vi "Modbus Samsung.vi"(5 "address":string, 6 "# Racks":i32=1, 7 "port (502)":u16=502, 8 "Error In":errorcluster, 10 "ES Reset":bool=TRUE, 11 "ES ON Array":bool[](array[boolean])) -> (0 "Error Out":errorcluster, 1 "Current Limit Parameters Out":T5 {"Min Cell Voltage Actual Value" format="%#.2f"; "Max Cell Voltage Actual Value" format="%#.2f"}, 2 "Energy Storage String Data Out":T3, 3 "Energy Storage System Data Out":T1={"Voltage"=0.0, "Current"=0.0, "SOC Avg"=0.0, "Faults"=0, "Alarms"=0, "# Strings"=0, "Max Temp"=0, "Min Temp"=0, "Max Cell Voltage"=0.0, "Min Cell Voltage"=0.0, "Energy Capacity"=0.0, "Energy Remaining"=0.0, "SOC Min"=0.0, "SOC Max"=0.0, "ES Fault"=FALSE, "String Select"=enum."3 Strings", "ES Com Fault"=FALSE, "SOH Avg"=0.0}, 4 "TCP Master Ref Out":refnum<class "Modbus Master.lvclass">)   [LabVIEW 2014]
uses:
  Controls/ModbusState.ctl
  <vilib>/Modbus/master/Modbus Master.lvclass
  Controls/Current Limit Parameters.ctl
  Controls/ES String Array.ctl
  Controls/ES String Data.ctl
  Controls/ES System Data.ctl
  Controls/StringSelector.ctl
  <vilib>/Modbus/master/Create Master Instance (TCP).vi
panel:
  out "Modbus State Out":T6
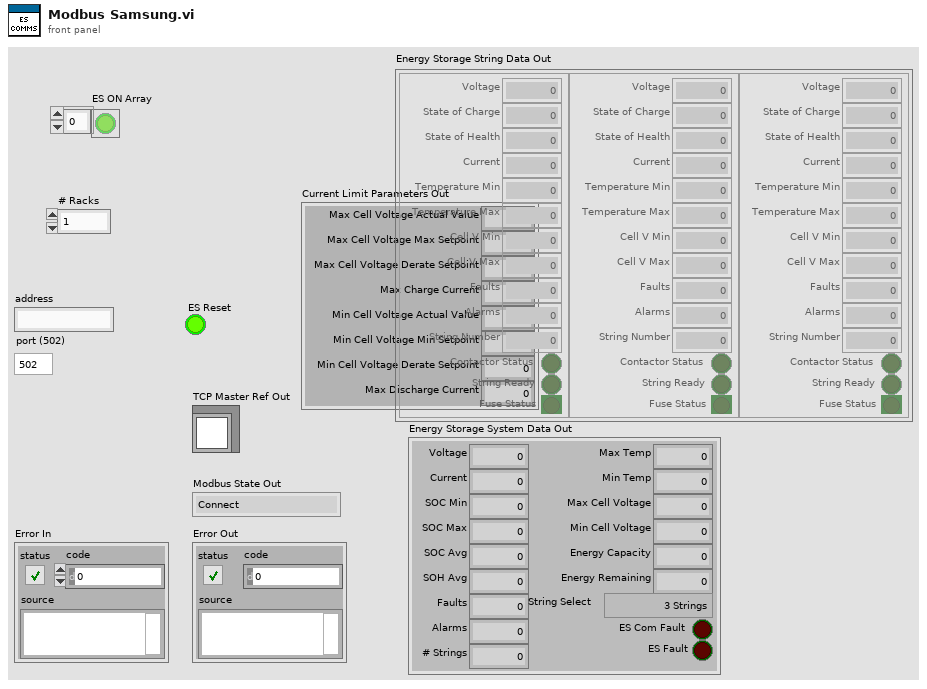
[diagram p1: front panel]
types:
  T1 = typedef "ES System Data.ctl" = cluster{"Voltage":sgl, "Current":sgl, "SOC Avg":sgl, "Faults":u16, "Alarms":u16, "# Strings":u16, "Max Temp":i16, "Min Temp":i16, "Max Cell Voltage":sgl, "Min Cell Voltage":sgl, "Energy Capacity":sgl, "Energy Remaining":sgl, "SOC Min":sgl, "SOC Max":sgl, "ES Fault":bool, "String Select":T2, "ES Com Fault":bool, "SOH Avg":sgl}
  T2 = typedef "StringSelector.ctl" = enum16{"1 String (1)", "1 String (2)", "1 String (3)", "2 Strings (1 2)", "2 Strings (2 3)", "2 Strings (1 3)", "3 Strings"}
  T3 = typedef "ES String Array.ctl" = T4[]
  T4 = typedef "ES String Data.ctl" = cluster{"Voltage":sgl, "State of Charge":sgl, "Current":sgl, "Temperature Min":i16, "Temperature Max":i16, "Faults":u16, "Alarms":u16, "String Number":u16, "Contactor Status":bool, "String Ready":bool, "Fuse Status":bool, "Cell V Max":dbl, "Cell V Min":dbl, "State of Health":sgl}
  T5 = typedef "Current Limit Parameters.ctl" = cluster{"Max Cell Voltage Max Setpoint":dbl, "Max Cell Voltage Actual Value":dbl, "Max Cell Voltage Derate Setpoint":dbl, "Max Charge Current":dbl, "Min Cell Voltage Min Setpoint":dbl, "Min Cell Voltage Actual Value":dbl, "Min Cell Voltage Derate Setpoint":dbl, "Max Discharge Current":dbl}
  T6 = typedef "ModbusState.ctl" = enum16{"Connect", "Disconnect", "Set Basic Objects", "Get Basic Objects", "Read", "Write", "Read/Write"}
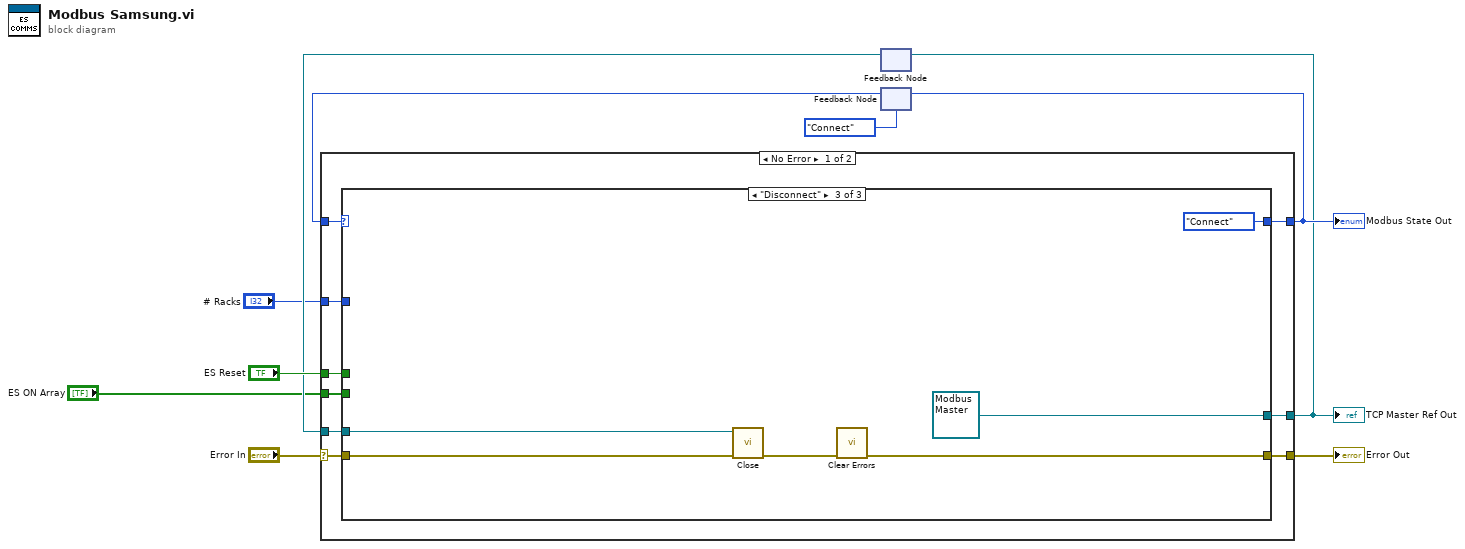
[diagram p0: block diagram]
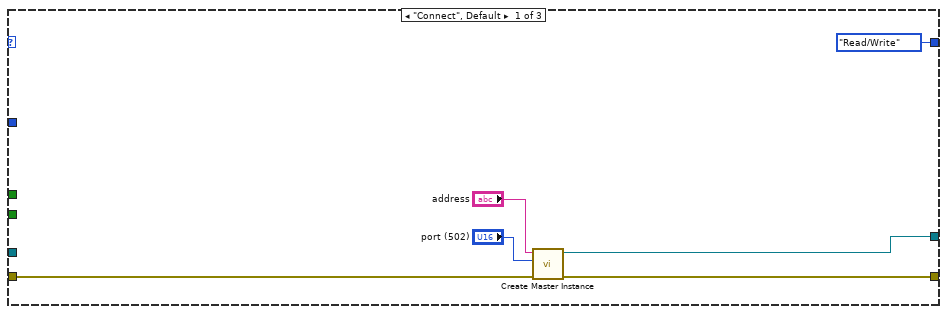
[diagram p2: hidden frame]
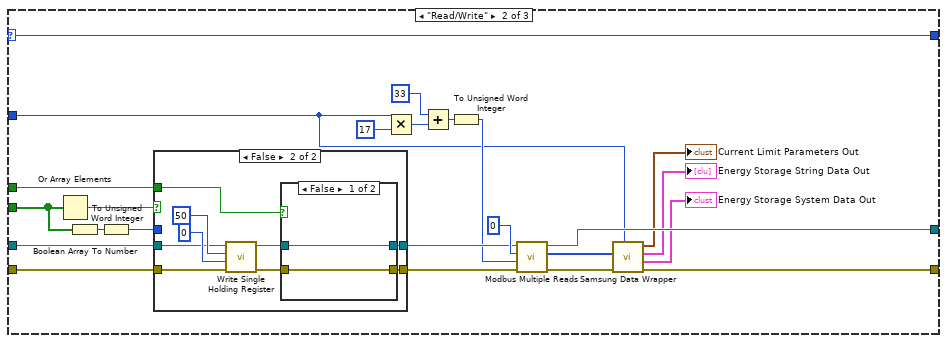
[diagram p3: hidden frame]
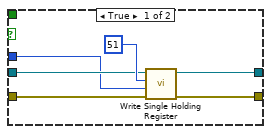
[diagram p4: hidden frame]
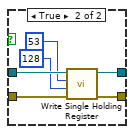
[diagram p5: hidden frame]
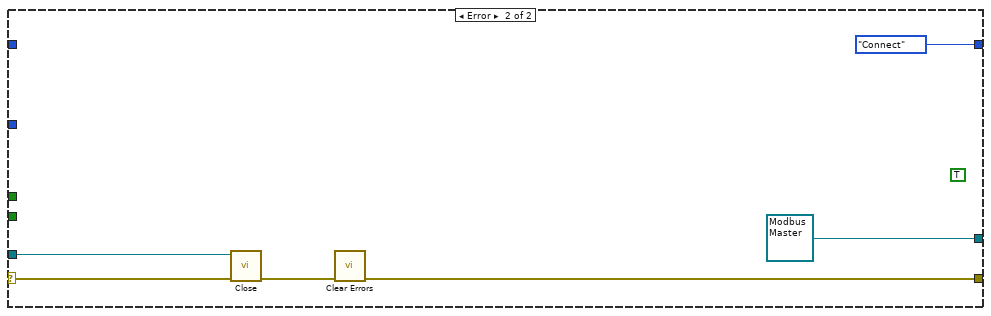
[diagram p6: hidden frame]
diagram:
  n1 = feedback #1() -> (w3:refnum<class "Modbus Master.lvclass">)  [unwired: 1 in]
  n2 = feedback #2(ModbusState."Connect" ("Modbus State In")) -> (w5:T6)
  n3 = case shown="No Error" "Error In" {
    selector: "Error In" -> [w18 w80]
    tunnel: [w15 w79] -> w9
    tunnel: w5 -> [w19 _]
    tunnel: [w17 refnum<class "Modbus Master.lvclass"> refnum ("TCP master instance")] -> w4
    tunnel: w3 -> [w16 w82]
    tunnel: [w14 ModbusState."Connect" ("Modbus State In")] -> w7
    tunnel: "ES Reset" -> [w13 _]
    tunnel: "ES ON Array" -> [w12 _]
    tunnel: "# Racks" -> [w11 _]
    frame No Error {
      n4 = case shown="\"Disconnect\"" w19 {
        selector: w19 -> [_ w47 _]
        tunnel: w18 -> [w25 w40 w77]
        tunnel: [w21 w49 refnum<class "Modbus Master.lvclass"> refnum ("TCP master instance")] -> w17
        tunnel: w16 -> [_ w39 w76]
        tunnel: [w22 w45 w75] -> w15
        tunnel: [ModbusState."Read/Write" ("Modbus State In") w47 ModbusState."Connect" ("Modbus State In")] -> w14
        tunnel: w13 -> [_ w38 _]
        tunnel: w12 -> [_ w34 _]
        tunnel: w11 -> [_ w26 _]
        frame "Connect", Default {
          n5 = call-poly <vilib>:"Create Master Instance.vi"("error in (no error)"=w25, "port (502)"="port (502)", "address"="address") -> ("error out"=w22:errorcluster, "TCP master instance"=w21:refnum<class "Modbus Master.lvclass">)  [unwired: 7 in]
        }
        frame "Read/Write" {
          n6 = Or Array Elements(Boolean array=w34) -> (logical OR=w35:bool)
          n7 = Boolean Array To Number(Boolean array=w34) -> (number=w33:u32)
          n8 = To Unsigned Word Integer(number=w33) -> (unsigned 16bit integer=w32:u16)
          n9 = case shown="False" w35 {
            tunnel: w40 -> [w54 w60]
            tunnel: w39 -> [w51 w57]
            tunnel: w38 -> [_ w64]
            tunnel: [w53 w63] -> w37
            tunnel: [w52 w62] -> w36
            tunnel: w32 -> [w50 _]
            frame True {
              n10 = call-dynamic "Write Single Holding Register.vi"("error in (no error)"=w54, "holding register value"=w50, "address"=u16 51, "Modbus master in"=w51) -> ("error out"=w53:errorcluster, "Modbus master out"=w52:refnum<class "Modbus Master.lvclass">)  [unwired: 6 in]
            }
            frame False {
              n11 = call-dynamic "Write Single Holding Register.vi"("error in (no error)"=w60, "holding register value"=u16 0, "address"=u16 50, "Modbus master in"=w57) -> ("error out"=w59:errorcluster, "Modbus master out"=w56:refnum<class "Modbus Master.lvclass">)  [unwired: 6 in]
              n12 = case shown="False" w64 {
                tunnel: w59 -> [w66 w72]
                tunnel: w56 -> [w65 w70]
                tunnel: [w66 w71] -> w63
                tunnel: [w65 w69] -> w62
                frame False {
                }
                frame True {
                  n13 = call-dynamic "Write Single Holding Register.vi"("error in (no error)"=w72, "holding register value"=u16 128, "address"=u16 53, "Modbus master in"=w70) -> ("error out"=w71:errorcluster, "Modbus master out"=w69:refnum<class "Modbus Master.lvclass">)  [unwired: 6 in]
                }
              }
            }
          }
          n14 = Multiply(x=w26, y=u8 17) -> (x*y=w30:i32)
          n15 = Add(x=u8 33, y=w30) -> (x+y=w28:i32)
          n16 = To Unsigned Word Integer(number=w28) -> (unsigned 16bit integer=w27:u16)
          n17 = call "Modbus Multiple Reads.vi"("Error In"=w37, "# elements to read"=w27, "Starting Address"=u16 0 ("starting address"), "Modbus Master In"=w36) -> ("Error Out"=w46:errorcluster, "register values"=w44:u16[], "Modbus Master Out"=w49:refnum<class "Modbus Master.lvclass">)  [unwired: 5 in]
          n18 = call "Samsung Data Wrapper.vi"("# Racks"=w26, "Error In"=w46, "Samsung Data In"=w44) -> ("Error Out"=w45:errorcluster, "Energy Storage System Data Out"=→"Energy Storage System Data Out":T1, "Energy Storage String Data Out"=→"Energy Storage String Data Out":T3, "Current Limit Parameters Out"=→"Current Limit Parameters Out":T5)  [unwired: 4 in, 1 out]
        }
        frame "Disconnect" {
          n19 = call-dynamic "Close.vi"("error in (no error)"=w77, "Modbus master in"=w76) -> ("error out"=w78:errorcluster)  [unwired: 9 in]
          n20 = call <vilib>:"Clear Errors.vi"("error in (no error)"=w78) -> ("error out"=w75:errorcluster)  [unwired: 5 in, 1 out]
        }
      }
    }
    frame Error {
      (unwired) TRUE
      n21 = call-dynamic "Close.vi"("error in (no error)"=w80, "Modbus master in"=w82) -> ("error out"=w83:errorcluster)  [unwired: 9 in]
      n22 = call <vilib>:"Clear Errors.vi"("error in (no error)"=w83) -> ("error out"=w79:errorcluster)  [unwired: 5 in, 1 out]
    }
  }
  "Error Out" <- w9
  "Modbus State Out" <- w7
  "TCP Master Ref Out" <- w4
  n23 = feedback-in #1(w4) -> ()
  n24 = feedback-in #2(w7) -> ()
